vi "Actor Core.vi"(8 "error in":errorcluster, 11 "Main View in":refnum<class "Main View.lvclass">) -> (0 "error out":errorcluster, 3 "Actor out":refnum<class "Actor.lvclass">)   [LabVIEW 2013, in "Main View.lvlib" / "Main View.lvclass"]
doc: "(<B>Filename</B>: Actor Framework.lvlib:Actor.lvclass:Actor Core.vi)\n\nReceives messages to the actor, reacts to them, and initiates any error handling that may shut the actor down.\n\nDescendant classes may override this VI to append parallel tasks for the actor to complete while it handles messages. Overrides use the Call Parent Method node."
uses:
  Main View.lvclass
  <vilib>/ActorFramework/Actor/Actor.lvclass
  Resources/UI Controls/Project Tile.ctl
  Resources/UI Controls/Sensor Tile.ctl
  <vilib>/ActorFramework/Actor/Actor.lvclass/Actor.ctl
  <vilib>/ActorFrameworkMVC/View Actor/View Actor.lvclass
  Main View.lvclass/Main View.ctl
  <vilib>/ActorFrameworkMVC/UI Controller Messages/Move Splitter Msg/Move Splitter Msg.lvclass/Move Splitter Msg.ctl
  <vilib>/ActorFramework/Message Enqueuer/Message Enqueuer.lvclass/Message Enqueuer.ctl
  <vilib>/Utility/miscctls.llb/LVPositionTypeDef.ctl
  <vilib>/ActorFrameworkMVC/UI Controller Messages/Move Subpanel Msg/Move Subpanel Msg.lvclass/Move Subpanel Msg.ctl
  <vilib>/ActorFrameworkMVC/UI Controller Messages/Insert Subpanel Msg/Insert Subpanel Msg.lvclass/Insert Subpanel Msg.ctl
  <vilib>/ActorFramework/Message Enqueuer/Enqueue.vi
  <vilib>/ActorFramework/Message Priority Queue/Priority Enqueue.vi
  <vilib>/ActorFrameworkMVC/UI Controller Messages/Move Splitter Msg/Move Splitter Msg.lvclass
  <vilib>/ActorFrameworkMVC/UI Controller Messages/Move Subpanel Msg/Move Subpanel Msg.lvclass
  <vilib>/ActorFrameworkMVC/UI Controller Messages/Insert Subpanel Msg/Insert Subpanel Msg.lvclass
  Models/Project Model Messages/Initialize Page Number Msg/Initialize Page Number Msg.lvclass
  Models/Project Model Messages/Preview Project Msg/Preview Project Msg.lvclass
  Models/Project Model Messages/Update Tiles Info Msg/Update Tiles Info Msg.lvclass
  Models/Project Model Messages/Update Previous Button Visibility Msg/Update Previous Button Visibility Msg.lvclass
  Models/Project Model Messages/Update Next Button Visibility Msg/Update Next Button Visibility Msg.lvclass
  Models/Sensor Model Messages/Initialize Page Number Msg/Initialize Page Number Msg.lvclass
  Models/Sensor Model Messages/Preview Sensor Msg/Preview Sensor Msg.lvclass
  Models/Sensor Model Messages/Update Tiles Info Msg/Update Tiles Info Msg.lvclass
  Models/Sensor Model Messages/Update Previous Button Visibility Msg/Update Previous Button Visibility Msg.lvclass
  Models/Sensor Model Messages/Update Next Button Visibility Msg/Update Next Button Visibility Msg.lvclass
  <vilib>/ActorFrameworkMVC/UI Controller Messages/Get Model Actor Enqueuer Msg/Get Model Actor Enqueuer Msg.lvclass
panel:
  out "Sensor Number":i32
  out "Project Number":i32
  in  "Sensor Tile":T1
  in  "Project Tile":T2
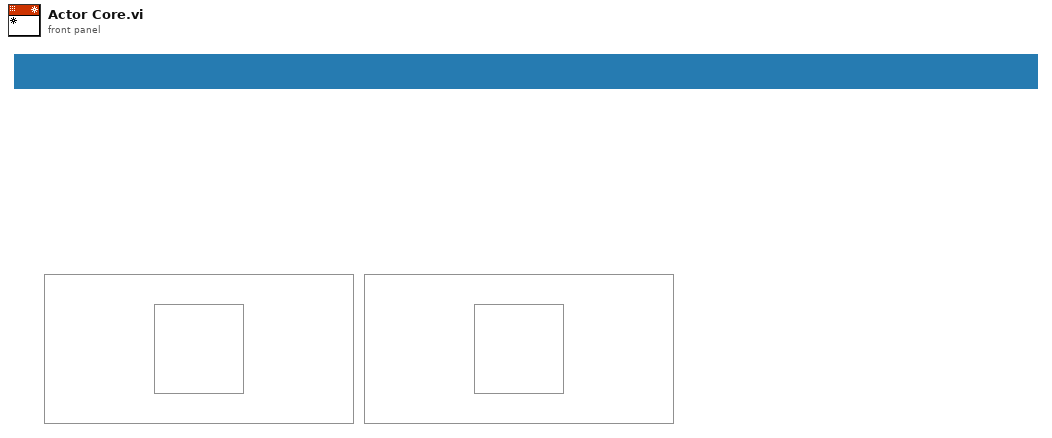
[diagram p1: front panel]
types:
  T1 = typedef "Sensor Tile.ctl" = bool
  T2 = typedef "Project Tile.ctl" = bool
  T3 = typedef "Main View.lvlib/Main View.lvclass/Events.ctl" = cluster{"Update Project Number":refnum<user-event>, "Update Sensor Number":refnum<user-event>}
  T4 = typedef "LVPositionTypeDef.ctl" = cluster{"Left":i32, "Top":i32}
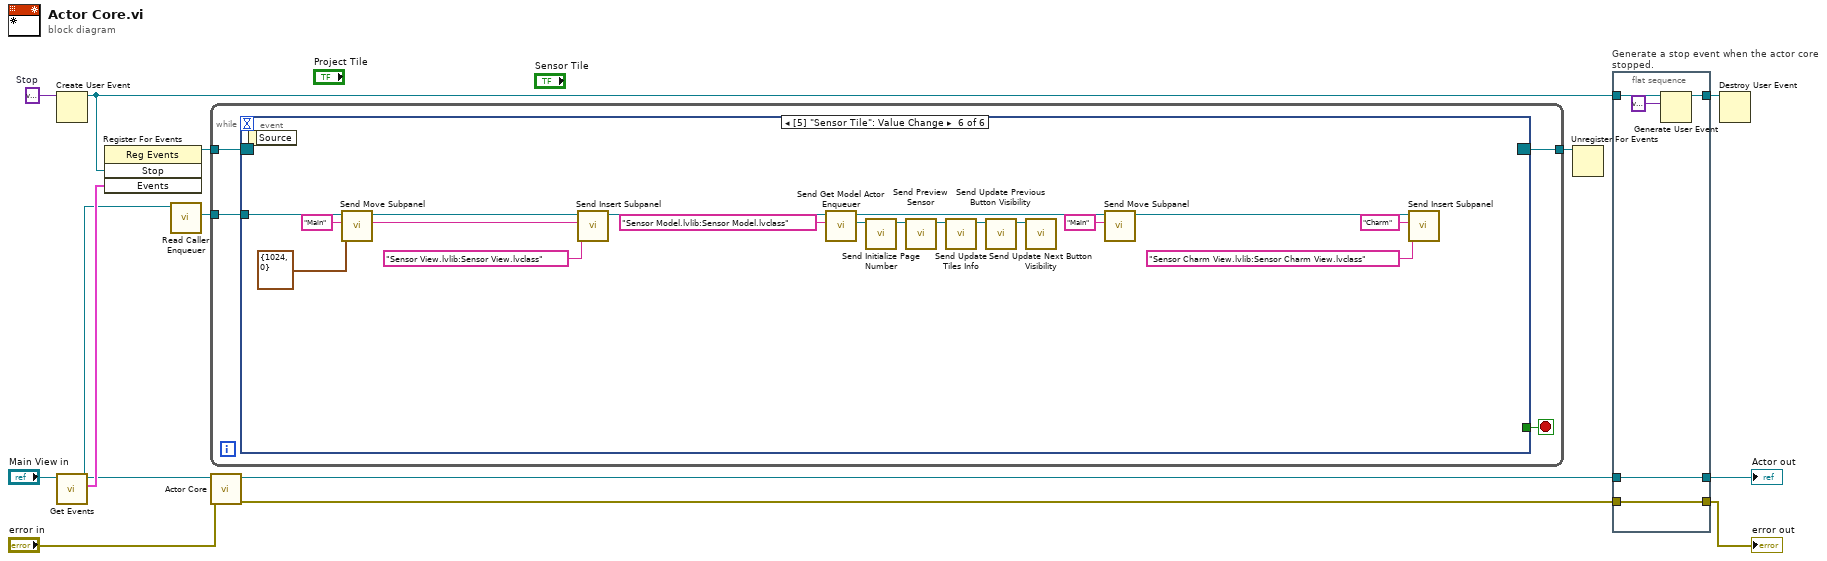
[diagram p0: block diagram]
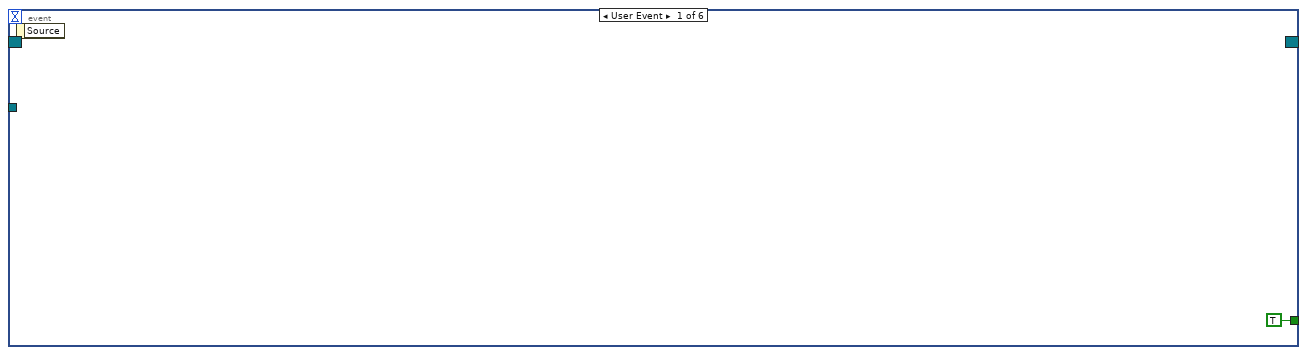
[diagram p2: hidden frame]
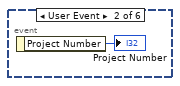
[diagram p3: hidden frame]
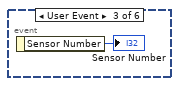
[diagram p4: hidden frame]
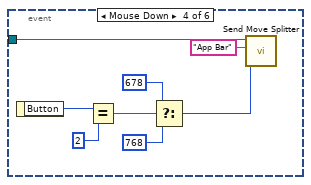
[diagram p5: hidden frame]
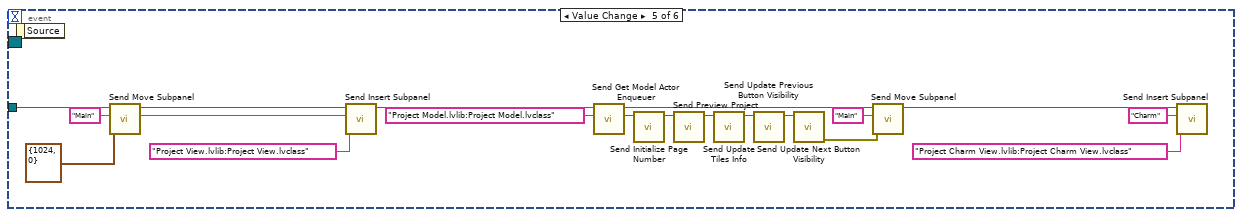
[diagram p6: hidden frame]
diagram:
  w14 = variant  # Stop
  n1 = Create User Event(user event datatype=w14) -> (user event=w5:refnum<user-event>)  [unwired: 1 in, 1 out]
  n2 = call "Get Events.vi"("Main View in"="Main View in") -> ("Events"=w4:T3, "Main View out"=w2:refnum<class "Main View.lvclass">)  [unwired: 9 in]
  n3 = register-events(w5, w4) -> (reference out=w6:refnum<event-registration>)  [unwired: 2 in, 1 out]
  n4 = call <vilib>:"Read Caller Enqueuer.vi"("Actor"=w2) -> ("Caller Enqueuer"=w1:refnum<class "Message Enqueuer.lvclass">)  [unwired: 10 in]
  n5 = while {
    tunnel: [w18] -> w3
    tunnel: w6 -> [w16]
    tunnel: w1 -> [w15]
    stop <- w17 stop-if-true
    n6 = event shown="[5] \"Sensor Tile\": Value Change" {
      selector: w16 -> [_ _ _ _ _ _]
      dyn-events: [_ _ _ _ _ _] -> w18
      timeout: _ -> [_ _ _ _ _ _]
      tunnel: [TRUE _ _ _ _ _] -> w17
      tunnel: w15 -> [_ _ _ w28 w47 w64]
      event User Event {
        n7 = event-data() -> ()  [unwired: 1 in, 1 out]
      }
      event User Event {
        n8 = event-data() -> ("Project Number"=→"Project Number":i32)  [unwired: 1 in]
      }
      event User Event {
        n9 = event-data() -> ("Sensor Number"=→"Sensor Number":i32)  [unwired: 1 in]
      }
      event Mouse Down {
        n10 = event-data() -> ("Button"=w27:u16)  [unwired: 1 in]
        n11 = Equal?(x=w27, y=u16 2) -> (x = y?=w25:bool)
        n12 = Select(t=678 ("Splitter Position"), s=w25, f=768 ("Splitter Position")) -> (s? t:f=w22:i32)
        n13 = call <vilib>:"Send Move Splitter.vi"("Splitter Position"=w22, "Splitter Name"="App Bar", "Message Enqueuer"=w28) -> ()  [unwired: 7 in, 2 out]
      }
      event Value Change {
        w43 = "Main" ("Subpanel Name")
        n14 = event-data() -> ()  [unwired: 1 in, 1 out]
        n15 = call <vilib>:"Send Move Subpanel.vi"("Position (0,0)"=T4 {"Left"=1024, "Top"=0}, "Subpanel Name"=w43, "Message Enqueuer"=w47) -> ("Message Enqueuer out"=w46:refnum<class "Message Enqueuer.lvclass">)  [unwired: 7 in, 1 out]
        n16 = call <vilib>:"Send Insert Subpanel.vi"("View Name"="Project View.lvlib:Project View.lvclass" ("Subpanel Name"), "Subpanel Name"=w43, "Message Enqueuer"=w46) -> ("Message Enqueuer out"=w39:refnum<class "Message Enqueuer.lvclass">)  [unwired: 7 in, 1 out]
        n17 = call <vilib>:"Send Get Model Actor Enqueuer.vi"("Model Name"="Project Model.lvlib:Project Model.lvclass", "Message Enqueuer in"=w39) -> ("Reply"=w41:refnum<class "Message Enqueuer.lvclass">, "Message Enqueuer out"=w38:refnum<class "Message Enqueuer.lvclass">)  [unwired: 6 in, 2 out]
        n18 = call "Send Initialize Page Number.vi"("Message Enqueuer"=w41) -> ("Message Enqueuer out"=w33:refnum<class "Message Enqueuer.lvclass">)  [unwired: 9 in, 1 out]
        n19 = call "Send Preview Project.vi"("Message Enqueuer"=w33) -> ("Message Enqueuer out"=w40:refnum<class "Message Enqueuer.lvclass">)  [unwired: 9 in, 1 out]
        n20 = call "Send Update Tiles Info.vi"("Message Enqueuer"=w40) -> ("Message Enqueuer out"=w36:refnum<class "Message Enqueuer.lvclass">)  [unwired: 9 in, 1 out]
        n21 = call "Send Update Previous Button Visibility.vi"("Message Enqueuer"=w36) -> ("Message Enqueuer out"=w35:refnum<class "Message Enqueuer.lvclass">)  [unwired: 9 in, 1 out]
        n22 = call "Send Update Next Button Visibility.vi"("Message Enqueuer"=w35) -> ("error out"=w34:errorcluster)  [unwired: 9 in, 1 out]
        n23 = call <vilib>:"Send Move Subpanel.vi"("error in (no error)"=w34, "Subpanel Name"="Main", "Message Enqueuer"=w38) -> ("Message Enqueuer out"=w32:refnum<class "Message Enqueuer.lvclass">)  [unwired: 7 in, 1 out]
        n24 = call <vilib>:"Send Insert Subpanel.vi"("View Name"="Project Charm View.lvlib:Project Charm View.lvclass", "Subpanel Name"="Charm", "Message Enqueuer"=w32) -> ()  [unwired: 7 in, 2 out]
      }
      event Value Change {
        w60 = "Main" ("Subpanel Name")
        n25 = event-data() -> ()  [unwired: 1 in, 1 out]
        n26 = call <vilib>:"Send Move Subpanel.vi"("Position (0,0)"=T4 {"Left"=1024, "Top"=0}, "Subpanel Name"=w60, "Message Enqueuer"=w64) -> ("Message Enqueuer out"=w63:refnum<class "Message Enqueuer.lvclass">)  [unwired: 7 in, 1 out]
        n27 = call <vilib>:"Send Insert Subpanel.vi"("View Name"="Sensor View.lvlib:Sensor View.lvclass" ("Subpanel Name"), "Subpanel Name"=w60, "Message Enqueuer"=w63) -> ("Message Enqueuer out"=w58:refnum<class "Message Enqueuer.lvclass">)  [unwired: 7 in, 1 out]
        n28 = call <vilib>:"Send Get Model Actor Enqueuer.vi"("Model Name"="Sensor Model.lvlib:Sensor Model.lvclass", "Message Enqueuer in"=w58) -> ("Reply"=w54:refnum<class "Message Enqueuer.lvclass">, "Message Enqueuer out"=w57:refnum<class "Message Enqueuer.lvclass">)  [unwired: 6 in, 2 out]
        n29 = call "Send Initialize Page Number.vi"("Message Enqueuer"=w54) -> ("Message Enqueuer out"=w53:refnum<class "Message Enqueuer.lvclass">)  [unwired: 9 in, 1 out]
        n30 = call "Send Preview Sensor.vi"("Message Enqueuer"=w53) -> ("Message Enqueuer out"=w52:refnum<class "Message Enqueuer.lvclass">)  [unwired: 9 in, 1 out]
        n31 = call "Send Update Tiles Info.vi"("Message Enqueuer"=w52) -> ("Message Enqueuer out"=w51:refnum<class "Message Enqueuer.lvclass">)  [unwired: 9 in, 1 out]
        n32 = call "Send Update Previous Button Visibility.vi"("Message Enqueuer"=w51) -> ("Message Enqueuer out"=w50:refnum<class "Message Enqueuer.lvclass">)  [unwired: 9 in, 1 out]
        n33 = call "Send Update Next Button Visibility.vi"("Message Enqueuer"=w50) -> ()  [unwired: 9 in, 2 out]
        n34 = call <vilib>:"Send Move Subpanel.vi"("Subpanel Name"="Main", "Message Enqueuer"=w57) -> ("Message Enqueuer out"=w55:refnum<class "Message Enqueuer.lvclass">)  [unwired: 8 in, 1 out]
        n35 = call <vilib>:"Send Insert Subpanel.vi"("View Name"="Sensor Charm View.lvlib:Sensor Charm View.lvclass", "Subpanel Name"="Charm", "Message Enqueuer"=w55) -> ()  [unwired: 7 in, 2 out]
      }
    }
  }
  n36 = call-parent "Actor Core.vi"("error in"="error in", "View Actor in"=w2) -> ("error out"=w9:errorcluster, "Actor out"=w10:refnum<class "Actor.lvclass">)  [unwired: 8 in]
  n37 = Unregister For Events(event registration refnum=w3) -> ()  [unwired: 1 in, 1 out]
  n38 = flat-sequence "Generate a stop event when the actor core stopped." {
    tunnel: w5 -> [w69]
    tunnel: [w67] -> w13
    tunnel: w10 -> [w66]
    tunnel: w9 -> [w65]
    tunnel: [w66] -> w8
    tunnel: [w65] -> w7
    frame #0 {
      n39 = Generate User Event(user event=w69, event data cluster=variant ("event data")) -> (user event out=w67:refnum<user-event>)  [unwired: 2 in, 1 out]
    }
  }
  n40 = Destroy User Event(user event=w13) -> ()  [unwired: 1 in, 1 out]
  "error out" <- w7
  "Actor out" <- w8
